vi "JL - Verify Scroll.vi"(0 "GEA2 Reference In":refnum<k24>, 1 "Timeout (sec)":dbl=3.0, 2 "Scroll Text":string, 11 "Error In":errorcluster) -> (4 "GEA2 Reference Out":refnum<k24>, 6 "Pass/Fail?":bool, 8 "Report Text":string, 15 "Error Out":errorcluster)   [LabVIEW 2016]
doc: "This VI is used to verify SSD scrolling messages on the HEUI."
uses:
  Q:/Common/DLLs/GEA3/GeaCommunication.dll
  Common/DLLs/GEA3/GeaCommunication.dll
  Common/LabVIEW GEA2 Toolkit/LabVIEW_GEA2_Toolkit.lvlibp/type defs/Source_Destination.ctl
  Common/LabVIEW GEA2 Toolkit/LabVIEW_GEA2_Toolkit.lvlibp/type defs/ERD Read Data In.ctl
  Common/LabVIEW GEA2 Toolkit/LabVIEW_GEA2_Toolkit.lvlibp/type defs/Data Type.ctl
  Common/LabVIEW GEA2 Toolkit/LabVIEW_GEA2_Toolkit.lvlibp
panel:
  in  "Standalone":bool
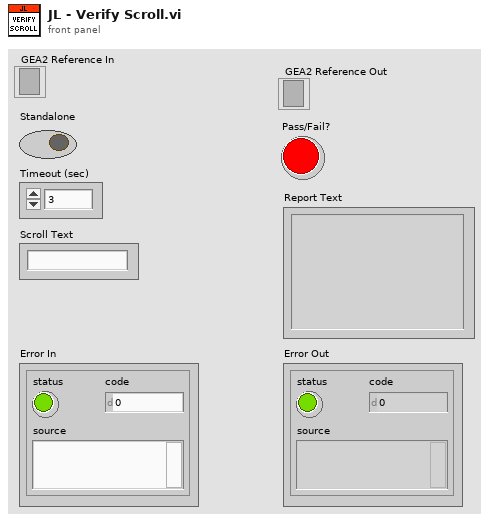
[diagram p1: front panel]
types:
  T1 = typedef "LabVIEW_GEA2_Toolkit.lvlibp/ERD Read Data In.ctl" = cluster{"ERD Number":u16, "Data Type":T2}
  T2 = typedef "LabVIEW_GEA2_Toolkit.lvlibp/Data Type.ctl" = enum16{"string", "boolean", "uint8_t", "uint16_t", "uint32_t", "uint64_t", "int8_t", "int16_t", "int32_t", "int64_t"}
  T3 = typedef "LabVIEW_GEA2_Toolkit.lvlibp/Source_Destination.ctl" = cluster{"Source":u8, "Destination":u8}
  T4 = typedef "LabVIEW_GEA2_Toolkit.lvlibp/ERD Read Data Out.ctl" = cluster{"ERD Number":u16, "Data":string}
  T5 = typedef "UI_LEDs.ctl" = cluster{"Z301 - Encoder 0":bool, "Z302 - Encoder 13":bool, "Z303 - Encoder 12":bool, "Z304 - Encoder 11":bool, "Z305 - Encoder 10":bool, "Z306 - Encoder 09":bool, "Z307 - Encoder 08":bool, "Z308 - Encoder 07":bool, "Z309 - Encoder 06":bool, "Z310 - Encoder 05":bool, "Z311 - Encoder 04":bool, "Z312 - Encoder 03":bool, "Z313 - Encoder 02":bool, "Z314 - Encoder 01":bool, "Z315 - Unpopulated":bool, "Z316 - Unpopulated":bool, "Z317 - SSD1:A":bool, "Z318 - SSD1:B":bool, "Z319 - SSD1:G":bool, "Z320 - SSD1:C":bool, "Z321 - SSD1:D":bool, "Z322 - SSD1:E":bool, "Z323 - SSD1:F":bool, "Z324 - Pause 1":bool, "Z325 - Control Lock 1":bool, "Z326 - Sensing 1":bool, "Z327 - Clean Lint Filter 1":bool, "Z328 - Extra Status 1":bool, "Z329 - Extra Status 2":bool, "Z330 - Clean Lint Filter 2":bool, "Z331 -Sensing 2":bool, "Z332 - Unpopulated":bool, "Z333 - SSD2:A":bool, "Z334 - SSD2:B":bool, "Z335 - SSD2:G":bool, "Z345 - SSD2:C":bool, "Z336 - SSD2:D":bool, "Z337 - SSD2:E":bool, "Z338 - SSD2:F":bool, "Z339 - Pause 3":bool, "Z340 - Control Lock 3":bool, "Z353 - Sensing 3":bool, "Z342 - Clean Lint Filter 3":bool, "Z344 - Extra Status 3":bool, "Z346 - Extra Status 4":bool, "Z341 - Pause 2":bool, "Z343 - Control Lock 2":bool, "Z347 - Unpopulated":bool, "Z348 -My Cycle":bool, "Z349 - Delay Dry":bool, "Z350 - Volume":bool, "Z351 - Damp Alert":bool, "Z352 - Bar 1":bool, "Z354 - Bar 2":bool, "Z355 - Bar 3":bool, "Z356 - Bar 4":bool, "Z357 - Bar 5":bool, "Z358 - eDry":bool, "Z359 - Time Increment":bool, "Z360 - Time Decrement":bool, "Z361 - Extended Tumble":bool, "Z362 - Unpopulated":bool, "Z363 - Unpopulated":bool, "Z364 - Unpopulated":bool, "Z365 - Status 1":bool, "Z366 - Status 3":bool, "Z367 - Default Time 5":bool, "Z368 - Default Time 4":bool, "Z369 - Default Time 3":bool, "Z370 - Dry":bool, "Z371 - Status 2":bool, "Z372 -Default Time 2":bool, "Z373 - Default Time 1":bool, "Z374 - Unpopulated":bool, "Z375 - Default Time 0":bool, "Z376 - No Heat":bool, "Z377 - Unpopulated":bool, "Z378 - Unpopulated":bool, "Z379 - Unpopulated":bool, "Z380 - Unpopulated":bool, "Z381 - Status 4":bool, "Z382 - Status 6":bool, "Z383 - More Dry":bool, "Z384 - High":bool, "Z385 - Medium":bool, "Z386 -Low":bool, "Z387 - Status 5":bool, "Z388 - Less Dry":bool, "Z388 - Extra Low":bool, "Z390 - Unpopulated":bool, "Z391 - Damp":bool, "Z392 - Unpopulated":bool, "Z393 - Unpopulated":bool, "Z394 - Unpopulated":bool, "Z395 - Unpopulated":bool, "Z396 - Unpopulated":bool, "Z101 - unpop?":bool, "Z102 - Start/Pause":bool, "OFF - OFF":bool, "MAX - MAX":bool}
  T6 = typedef "JL Display.ctl" = cluster{"SSD":string, "Cycle Selection":T7, "Bar Selection":T8, "Temp Setting":T9, "Dryness Level":T10, "Time Setting":T11, "Dryer Status":T12, "Start/Pause":bool, "Pause":bool, "Control Lock":bool, "Sensing":bool, "Clean Filter":bool, "My Cycle":bool, "Delay Dry":bool, "Volume":bool, "Damp Alert":bool, "Ext Tumble":bool, "Decrement":bool, "Increment":bool, "eDry":bool, "Extra Status":bool}
  T7 = typedef "Cycle Selection Enum.ctl" = enum16{"Cycle 0", "Cycle 1", "Cycle 2", "Cycle 3", "Cycle 4", "Cycle 5", "Cycle 6", "Cycle 7", "Cycle 8", "Cycle 9", "Cycle 10", "Cycle 11", "Cycle 12", "Cycle 13", "Off", "*Invalid"}
  T8 = typedef "Bar Enum.ctl" = enum16{"Bar 1", "Bar 2", "Bar 3", "Bar 4", "Bar 5", "Off", "*Incorrect*"}
  T9 = typedef "Temp Setting Enum.ctl" = enum16{"Off", "No Heat", "Extra Low", "Low", "Medium", "High", "*Incorrect*"}
  T10 = typedef "Dryness Enum.ctl" = enum16{"Off", "Damp", "Less Dry", "Dry", "More Dry", "Extra Dry", "*Incorrect*"}
  T11 = typedef "Time Enum.ctl" = enum16{"Off", "Default Time 1", "Default Time 2", "Default Time 3", "Default Time 4", "Default Time 5", "*Incorrect*"}
  T12 = typedef "Status Enum.ctl" = enum16{"Status 1", "Status 2", "Status 3", "Status 4", "Status 5", "Status 6", "Off", "*Incorrect*"}
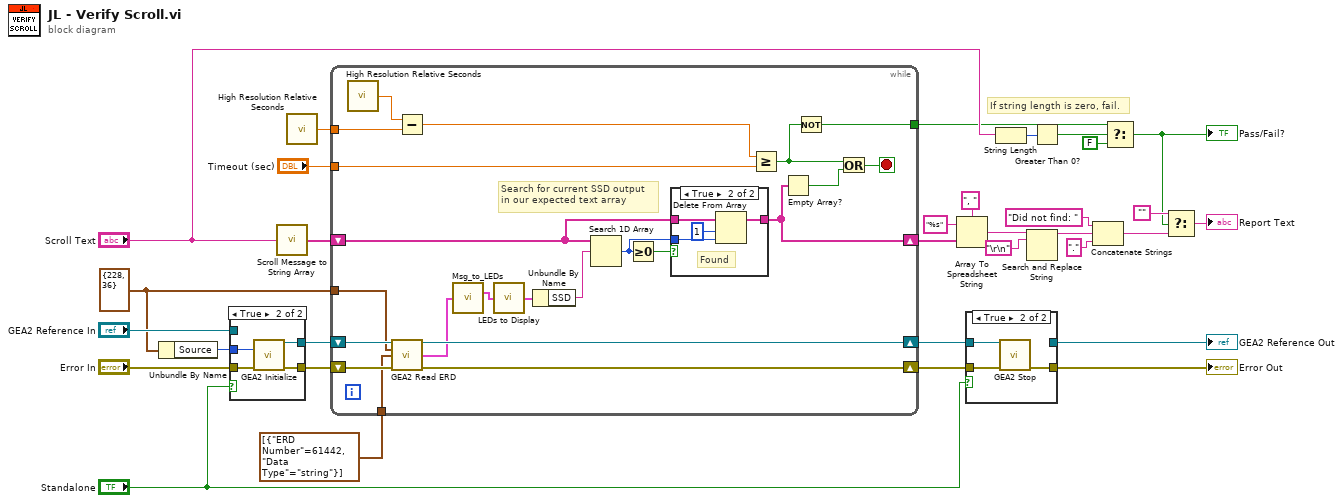
[diagram p0: block diagram]
diagram:
  w20 = T3 {"Source"=228, "Destination"=36} ("GEA Inputs")
  # "If string length is zero, fail."
  n1 = Unbundle By Name(w20) -> ("Source"=w31:u8)
  n2 = case shown="True" "Standalone" {
    tunnel: "Error In" -> [w34 w38]
    tunnel: w31 -> [_ w37]
    tunnel: [w33 w36] -> w27
    tunnel: [w34 w35] -> w26
    tunnel: "GEA2 Reference In" -> [w33 _]
    frame False {
    }
    frame True {
      n3 = call "GEA2 Initialize.vi"("Source Address"=w37, "error in"=w38) -> ("GEA2 Reference Out"=w36:refnum<k24>, "error out"=w35:errorcluster)  [unwired: 11 in, 1 out]
    }
  }
  n4 = call "Scroll Message to String Array.vi"("Scroll Text"="Scroll Text") -> ("Array"=w23:string[])  [unwired: 14 in]
  n5 = call <vilib>:"High Resolution Relative Seconds.vi"() -> ("relative seconds"=w21:dbl)
  n6 = while {
    tunnel: w21 -> [w59]
    tunnel: [w41] -> w2
    shift-right: [w55] -> w25
    shift-left: w27 -> [w52]
    shift-right: [w54] -> w24
    shift-left: w26 -> [w53]
    tunnel: T1[] [{"ERD Number"=61442, "Data Type"=enum."string"}] ("Read ERD List") -> [w51]
    shift-right: [w40] -> w16
    shift-left: w23 -> [w45]
    tunnel: w20 -> [w43]
    tunnel: "Timeout (sec)" -> [w42]
    stop <- w57 stop-if-true
    # "Search for current SSD output\nin our expected text array"
    n7 = call <vilib>:"High Resolution Relative Seconds.vi"() -> ("relative seconds"=w60:dbl)
    n8 = call "GEA2 Read ERD.vi"("GEA2 Reference In"=w52, "GEA Inputs"=w43, "Read ERD List"=w51, "Error In"=w53) -> ("GEA2 Reference Out"=w55:refnum<k24>, "ERD Data Out"=w39:T4[], "Error Out"=w54:errorcluster)  [unwired: 8 in, 1 out]
    n9 = Subtract(x=w60, y=w59) -> (x-y=w58:dbl)
    n10 = call "Msg_to_LEDs.vi"("ERD Data Out"=w39) -> ("Justice League UI"=w50:T5)  [unwired: 11 in, 3 out]
    n11 = call "LEDs to Display.vi"("Justice League UI"=w50) -> ("JL Display"=w49:T6)  [unwired: 14 in]
    n12 = Unbundle By Name(w49) -> ("SSD"=w48:string)
    n13 = Search 1D Array(1D array=w45, element=w48) -> (index of element=w46:i32)  [unwired: 1 in]
    n14 = Greater Or Equal To 0?(x=w46) -> (x >= 0?=w47:bool)
    n15 = case shown="True" w47 {
      tunnel: w46 -> [_ w64]
      tunnel: w45 -> [w61 w65]
      tunnel: [w61 w62] -> w40
      frame False {
        # "Not Found"
      }
      frame True {
        # "Found"
        n16 = Delete From Array(array=w65, length=1, index=w64) -> (array with subset deleted=w62:string[])  [unwired: 1 out]
      }
    }
    n17 = Greater Or Equal?(x=w58, y=w42) -> (x >= y?=w56:bool)
    n18 = Empty Array?(array=w40) -> (empty?=w44:bool)
    n19 = Not(x=w56) -> (.not. x?=w41:bool)
    n20 = Or(x=w56, y=w44) -> (x .or. y?=w57:bool)
  }
  n21 = Array To Spreadsheet String(delimiter (Tab)=", ", array=w16, 3:"%s" ("format string")) -> (spreadsheet string=w10:string)
  n22 = case shown="True" "Standalone" {
    tunnel: w24 -> [w67 w70]
    tunnel: [w67 w69] -> w12
    tunnel: w25 -> [w66 w68]
    tunnel: [w66 _] -> w28
    frame False {
    }
    frame True {
      n23 = call "GEA2 Stop.vi"("GEA2 Reference In"=w68, "Error In"=w70) -> ("Error Out"=w69:errorcluster)  [unwired: 13 in]
    }
  }
  "GEA2 Reference Out" <- w28
  "Error Out" <- w12
  n24 = String Length(string="Scroll Text") -> (length=w5:i32)
  n25 = Search and Replace String(input string=w10, search string="\r\n") -> (result string=w8:string)  [unwired: 6 in, 3 out]
  n26 = Greater Than 0?(x=w5) -> (x > 0?=w4:bool)
  n27 = Concatenate Strings("Did not find: " ("string"), w8, "." ("string")) -> (w7:string)
  n28 = Select(t=w2, s=w4, f=FALSE) -> (s? t:f=w3:bool)
  "Pass/Fail?" <- w3
  n29 = Select(t="", s=w3, f=w7) -> (s? t:f=→"Report Text":string)
